vi "Share Queue.vi"(8 "error in (no error)":errorcluster, 11 "Thread in":refnum<class "Thread.lvclass">) -> (0 "error out":errorcluster, 2 "Architecture.lvlib:Queue.lvclass":refnum<class "Queue.lvclass">, 3 "Thread out":refnum<class "Thread.lvclass">)   [LabVIEW 2013, in "Architecture.lvlib" / "Thread.lvclass"]
uses:
  Thread.lvclass
  Queue.lvclass
  Thread.lvclass/Thread.ctl
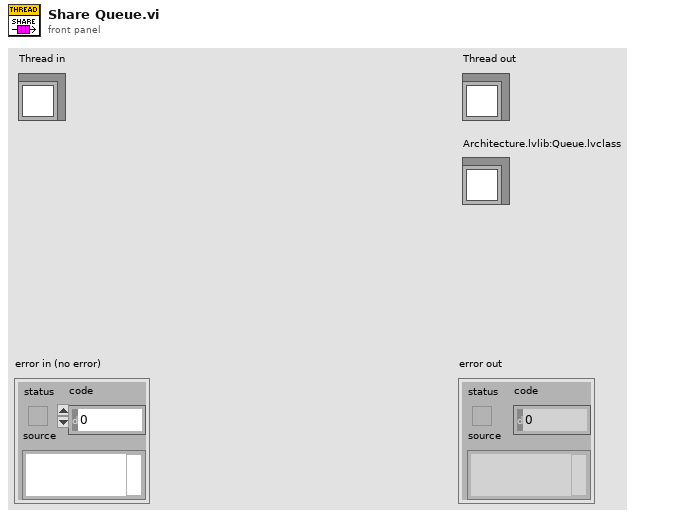
[diagram p1: front panel]
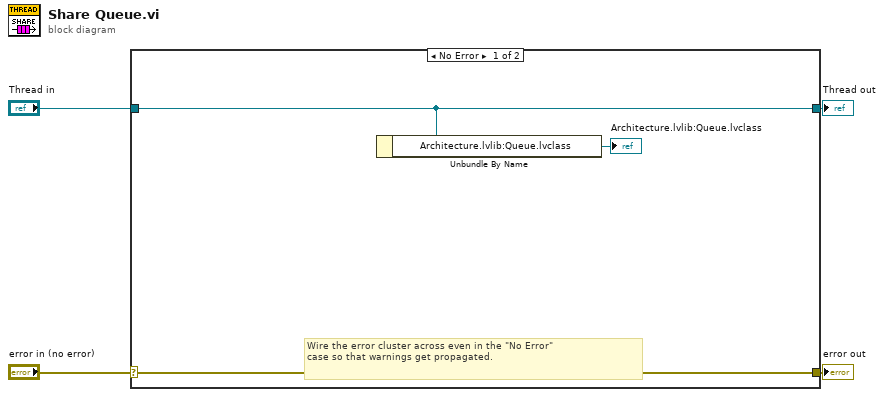
[diagram p0: block diagram]
diagram:
  n1 = case shown="No Error" "error in (no error)" {
    selector: "error in (no error)" -> [w7 w9]
    tunnel: [w7 w9] -> w3
    tunnel: [w6 w8] -> w1
    tunnel: "Thread in" -> [w6 w8]
    frame No Error {
      # "Wire the error cluster across even in the \"No Error\"\ncase so that warnings get propagated."
      n2 = Unbundle By Name(w6) -> ("Architecture.lvlib:Queue.lvclass"=→"Architecture.lvlib:Queue.lvclass":refnum<class "Queue.lvclass">)
    }
    frame Error {
    }
  }
  "error out" <- w3
  "Thread out" <- w1
